vi "Set-sequence.vi"(8 "error in (no error)":errorcluster, 9 "Sequence":refnum<class "Action-sequence.lvclass">, 10 "Motor index":i32, 11 "Object ref in":T1) -> (0 "error out":errorcluster, 3 "Object ref out":T1)   [LabVIEW 2013, in "PowderDeposition.lvlib" / "PD-Main.lvclass"]
uses:
  PD-Main.lvclass
  Object-reference.ctl
  Sequence/Action-sequence.lvclass
  PD-Main.lvclass/PD-Main.ctl
  Read Motor sequences.vi
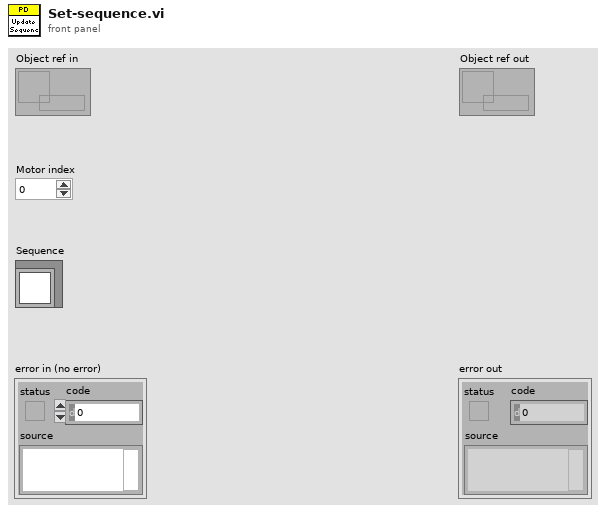
[diagram p1: front panel]
types:
  T1 = typedef "PowderDeposition.lvlib/PD-Main.lvclass/Object-reference.ctl" = refnum<data-value>
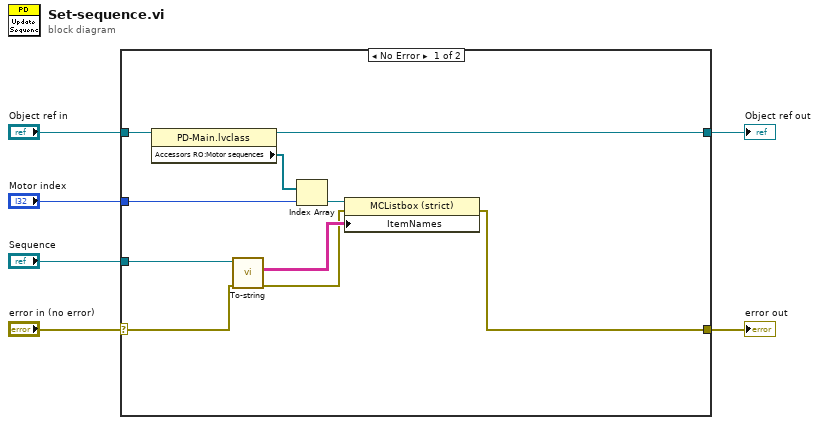
[diagram p0: block diagram]
diagram:
  n1 = case shown="No Error" "error in (no error)" {
    selector: "error in (no error)" -> [w10 w18]
    tunnel: [w7 w18] -> w5
    tunnel: [w15 w17] -> w3
    tunnel: "Object ref in" -> [w16 w17]
    tunnel: "Motor index" -> [w13 _]
    tunnel: "Sequence" -> [w11 _]
    frame No Error {
      n2 = property class="PD-Main.lvclass"(reference=w16) -> (reference out=w15:T1, "Accessors RO:Motor sequences"=w14:refnum<vi>[])  [unwired: 1 in, 1 out]
      n3 = call "To-string.vi"("error in (no error)"=w10, "Sequence in"=w11) -> ("error out"=w8:errorcluster, "Action string array"=w9:string[][])  [unwired: 7 in, 1 out]
      n4 = Index Array(array=w14, index=w13) -> (element=w12:refnum<vi>)
      n5 = property class="MCListbox (strict)"(reference=w12, error in=w8, "ItemNames"=w9) -> (error out=w7:errorcluster)  [unwired: 1 out]
    }
    frame Error {
    }
  }
  "error out" <- w5
  "Object ref out" <- w3
